vi "Debug_WFS_Tilt.vi"() -> ()   [LabVIEW 2014]
uses:
  AODAcq/AODAcq.lvclass
  <vilib>/rvi/interface/nirviReadWriteControl/nirviReadWriteControl.xnode
  FPGA_Control/AODRef.ctl
  <vilib>/DAQmx/write.llb/DAQmx Write (Analog DBL 1Chan 1Samp).vi
  <vilib>/Utility/file.llb/Write To Spreadsheet File (DBL).vi
  <vilib>/DAQmx/create/channels.llb/DAQmx Create Channel (AI-Voltage-Basic).vi
  <vilib>/DAQmx/read.llb/DAQmx Read (Analog 1D DBL NChan 1Samp).vi
  <vilib>/vision/driver/NI_Vision_Acquisition_Software.lvlib
  <vilib>/userdefined/High Color/IMAQdx.ctl
  <vilib>/vision/driver/IMAQdx.llb/IMAQdx Camera Control Mode.ctl
  <vilib>/rvi/errors/niLvFpgaAdjustHostInterfaceError.vi
  NiFpgaLv.dll
  <vilib>/Utility/error.llb/Error Cluster From Error Code.vi
  FPGA Bitfiles/AodScanner_FPGATarget_AODControl(FPGA)_TyJc9yYmyGA.lvbitx
panel:
  in  "Reps":i32=1
  out "Image":T1(plugin-control)
  in  "Measure centroid":bool
  out "Power":dbl
  in  "Save":bool
  in  "Range":dbl=214748364.8
  in  "stop":bool
  out "Corodinate Num":i32
  out "Num Coordinates":i32
  in  "NXHP":i32=10
  in  "NXLP":i32=10
  in  "NYHP":i32=10
  in  "NYLP":i32=10
  in  "Measure WFS":bool
  in  "Measure Power":bool
  in  "Hold time (ms)":u32=500
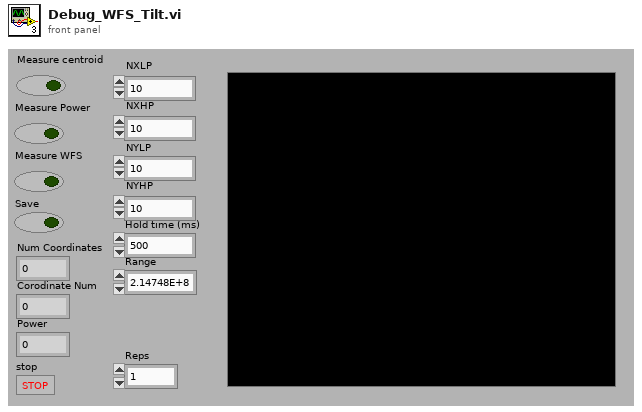
[diagram p1: front panel]
types:
  T1 = typedef "IMAQ Image.ctl" = refnum<image>
  T2 = typedef "NI_Vision_Acquisition_Software.lvlib/IMAQdx Camera Control Mode.ctl" = enum32{"Controller", "Listener"}
  T3 = typedef "IMAQdx.ctl" = refnum<k21>
  T4 = typedef "Image Type" = u32
  T5 = enum16{"Read", "Write", "ReadWrite", "BufferedRead", "BufferedReadWrite"}
  T6 = cluster{"XHP":i32, "XLP":i32, "YHP":i32, "YLP":i32}[]
  T7 = typedef "AODRef.ctl" = refnum<k20>
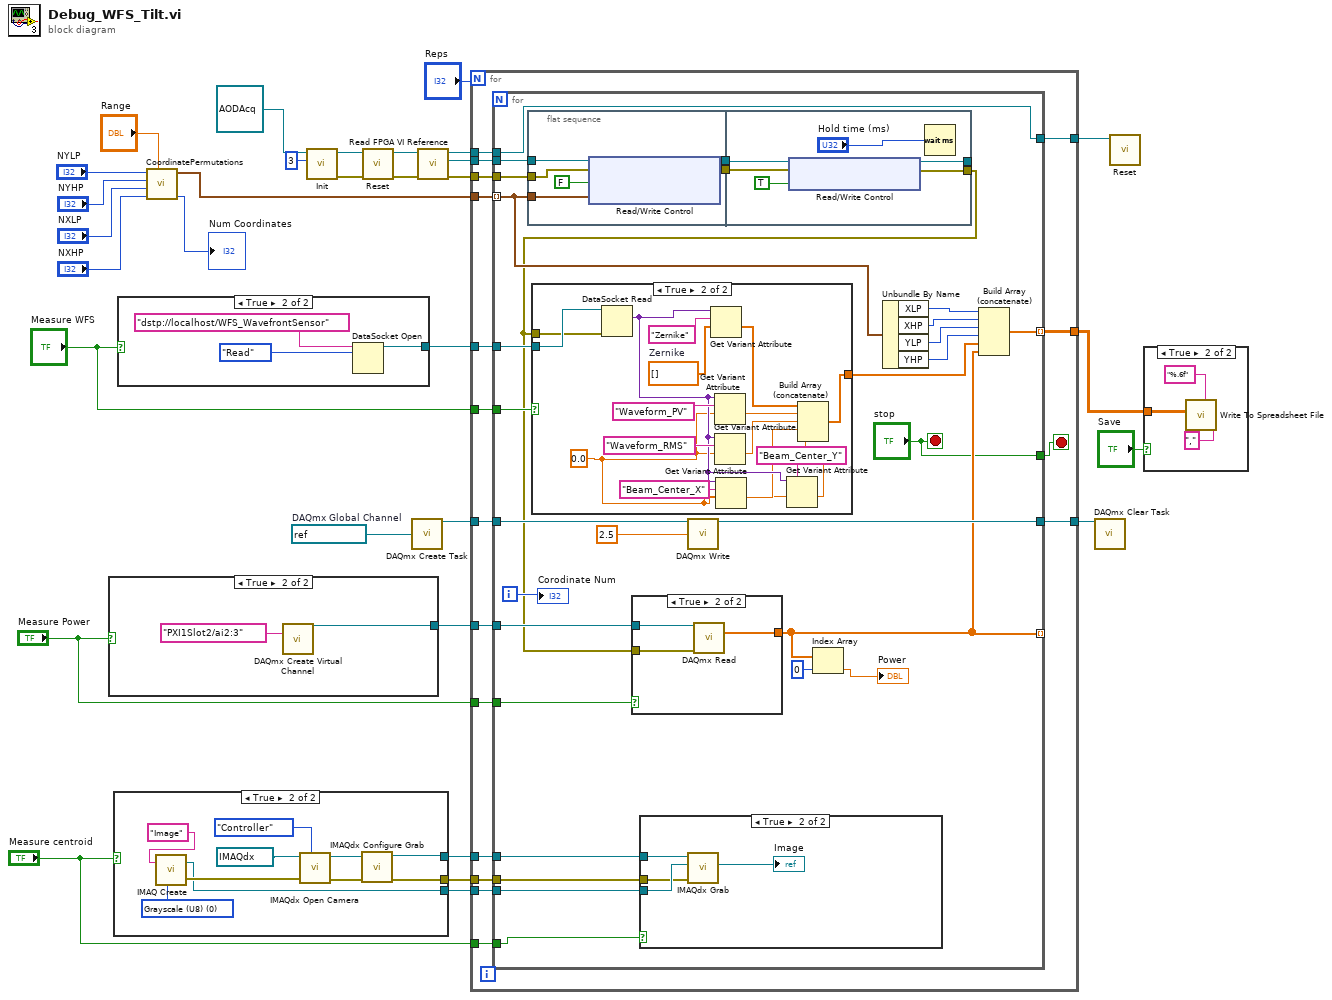
[diagram p0: block diagram]
diagram:
  w22 = refnum<k21> "AOD Gain"  # DAQmx Global Channel
  n1 = case shown="True" "Measure Power" {
    tunnel: [_ w32] -> w10
    frame False {
    }
    frame True {
      n2 = call-poly <vilib>:"DAQmx Create Virtual Channel.vi"("physical channels"=tag "PXI1Slot2/ai2:3") -> ("task out"=w32:refnum<k21>)  [unwired: 13 in, 1 out]
    }
  }
  n3 = case shown="True" "Measure centroid" {
    tunnel: [_ w35] -> w8
    tunnel: [_ w39] -> w6
    tunnel: [_ w34] -> w5
    frame False {
    }
    frame True {
      w41 = T4 0 items=["Grayscale (U8)", "Grayscale (I16)", "Grayscale (SGL)", "Complex (CSG)", "RGB (U32)", "HSL (U32)", "RGB (U64)", "Grayscale (U16)"] ("Image Type")
      n4 = call "IMAQ Create"("Image Name"="Image", "Image Type"=w41) -> ("New Image"=w39:T1, "error out"=w40:errorcluster)  [unwired: 3 in]
      n5 = call <vilib>:"IMAQdx Open Camera.vi"("Camera Control Mode"=IMAQdx_Camera_Control_Mode."Controller", "error in"=w40, "Session In"=T3 "cam1") -> ("error out"=w37:errorcluster, "Session Out"=w36:T3)  [unwired: 7 in]
      n6 = call <vilib>:"IMAQdx Configure Grab.vi"("error in"=w37, "Session In"=w36) -> ("error out"=w34:errorcluster, "Session Out"=w35:T3)  [unwired: 8 in]
    }
  }
  n7 = case shown="True" "Measure WFS" {
    tunnel: [_ w44] -> w23
    frame False {
    }
    frame True {
      n8 = DataSocket Open(10:T5."Read" ("mode"), 11:"dstp://localhost/WFS_WavefrontSensor" ("URL")) -> (3:w44:refnum<k13>)  [unwired: 2 in, 1 out]
    }
  }
  n9 = call "CoordinatePermutations.vi"("Range"="Range", "NXHP"="NXHP", "NXLP"="NXLP", "NYHP"="NYHP", "NYLP"="NYLP") -> ("Num Coordinates"=→"Num Coordinates":i32, "Coordinates"=w4:T6)  [unwired: 5 in]
  n10 = call-dynamic "Init.vi"("Channel"=i16 3, "AODAcq in"=refnum<class "AODAcq.lvclass"> refnum ("AODAcq.lvclass")) -> ("error out"=w29:errorcluster, "AODAcq out"=w30:refnum<class "AODAcq.lvclass">)  [unwired: 8 in]
  n11 = call-dynamic "Reset.vi"("error in (no error)"=w29, "AODAcq in"=w30) -> ("error out"=w26:errorcluster, "AODAcq out"=w28:refnum<class "AODAcq.lvclass">)  [unwired: 8 in]
  n12 = call <vilib>:"DAQmx Create Task.vi"("global virtual channels"=w22) -> ("task out"=w21:refnum<k21>)  [unwired: 4 in, 10 out]
  n13 = call-dynamic "Read FPGA VI Reference.vi"("error in (no error)"=w26, "AODAcq in"=w28) -> ("error out"=w25:errorcluster, "FPGA VI Reference"=w27:T7, "AODAcq out"=w19:refnum<class "AODAcq.lvclass">)  [unwired: 7 in]
  n14 = for {
    N: "Reps" -> [_]
    tunnel: w27 -> [w63]
    tunnel: w25 -> [w62]
    tunnel: "Measure WFS" -> [w61]
    tunnel: w23 -> [w60]
    tunnel: w21 -> [w59]
    tunnel: [w58] -> w20
    tunnel: w19 -> [w57]
    tunnel: [w56] -> w2
    tunnel: [w55] -> w12
    tunnel: w10 -> [w54]
    tunnel: "Measure Power" -> [w53]
    tunnel: w8 -> [w52]
    tunnel: "Measure centroid" -> [w51]
    tunnel: w6 -> [w50]
    tunnel: w5 -> [w49]
    tunnel: w4 -> [w48]
    stop <- w47 stop-if-true
    n15 = for {
      tunnel: w63 -> [w91]
      tunnel: w48 -> [w81] mode=indexing
      tunnel: w62 -> [w89]
      tunnel: w61 -> [w88]
      tunnel: w60 -> [w87]
      tunnel: w59 -> [w86]
      tunnel: [w84] -> w58
      tunnel: w57 -> [w83]
      tunnel: [w83] -> w56
      tunnel: [w75] -> w55 mode=indexing
      tunnel: w54 -> [w74]
      tunnel: w53 -> [w72]
      tunnel: [w71] -> _ mode=indexing
      tunnel: w52 -> [w67]
      tunnel: w51 -> [w68]
      tunnel: w50 -> [w66]
      tunnel: w49 -> [w65]
      tunnel: ["stop"] -> w47
      i -> [w82]
      stop <- "stop" stop-if-true
      n16 = flat-sequence {
        tunnel: w91 -> [w121]
        tunnel: [w119] -> w92
        tunnel: w81 -> [w118]
        tunnel: [w117] -> w90
        tunnel: w89 -> [w116]
        tunnel: w92 -> [w127]
        tunnel: w90 -> [w124]
        tunnel: [w123] -> w73
        tunnel: [w122] -> _
        frame #0 {
          n17 = xnode "Read/Write Control"("FPGA VI Reference In"=w121, "error in"=w116, "Debug.SetCoordinate"=FALSE, "Debug.Coordinate"=w118) -> ("FPGA VI Reference Out"=w119:T7, "error out"=w117:errorcluster)
        }
        frame #1 {
          n18 = xnode "Read/Write Control"("FPGA VI Reference In"=w127, "error in"=w124, "Debug.SetCoordinate"=TRUE) -> ("FPGA VI Reference Out"=w122:T7, "error out"=w123:errorcluster)
          n19 = Wait (ms)(milliseconds to wait="Hold time (ms)") -> ()  [unwired: 1 out]
        }
      }
      n20 = case shown="True" w88 {
        tunnel: w87 -> [_ w113]
        tunnel: w73 -> [_ w112]
        tunnel: [_ w106] -> w76
        frame False {
        }
        frame True {
          w101 = 0.0
          w115 = dbl[] []  # Zernike
          n21 = DataSocket Read(8:w112, 11:w113) -> (2:w105:variant)  [unwired: 3 in, 6 out]
          n22 = Get Variant Attribute(Variant=w105, name="Zernike", default value (empty Variant)=w115) -> (value=w109:dbl[])  [unwired: 1 in, 3 out]
          n23 = Get Variant Attribute(Variant=w105, name="Waveform_PV", default value (empty Variant)=w101) -> (value=w108:dbl)  [unwired: 1 in, 3 out]
          n24 = Get Variant Attribute(Variant=w105, name="Waveform_RMS", default value (empty Variant)=w101) -> (value=w107:dbl)  [unwired: 1 in, 3 out]
          n25 = Get Variant Attribute(Variant=w105, name="Beam_Center_X", default value (empty Variant)=w101) -> (value=w102:dbl)  [unwired: 1 in, 3 out]
          n26 = Get Variant Attribute(Variant=w105, name="Beam_Center_Y", default value (empty Variant)=w101) -> (value=w100:dbl)  [unwired: 1 in, 3 out]
          n27 = Build Array (concatenate)(w109, w108, w107, w102, w100) -> (w106:dbl[])
        }
      }
      n28 = case shown="True" w72 {
        tunnel: w74 -> [_ w99]
        tunnel: w73 -> [_ w98]
        tunnel: [_ w97] -> w71
        frame False {
        }
        frame True {
          n29 = call-poly <vilib>:"DAQmx Read.vi"("task/channels in"=w99, "error in"=w98) -> ("data"=w97:dbl[])  [unwired: 11 in, 2 out]
        }
      }
      n30 = case shown="True" w68 {
        tunnel: w67 -> [_ w96]
        tunnel: w66 -> [_ w94]
        tunnel: w65 -> [_ w93]
        frame False {
        }
        frame True {
          n31 = call <vilib>:"IMAQdx Grab.vi"("error in"=w93, "Image In"=w94, "Session In"=w96) -> ("Image Out"=→"Image":T1)  [unwired: 5 in, 3 out]
        }
      }
      n32 = call-poly <vilib>:"DAQmx Write.vi"("task/channels in"=w86, "data"=2.5) -> ("task out"=w84:refnum<k21>)  [unwired: 11 in, 2 out]
      n33 = Index Array(array=w71, index=0) -> (element=→"Power":dbl)
      n34 = Unbundle By Name(w81) -> ("XLP"=w80:i32, "XHP"=w79:i32, "YLP"=w78:i32, "YHP"=w77:i32)
      n35 = Build Array (concatenate)(w80, w79, w78, w77, w76, w71) -> (w75:dbl[])
      "Corodinate Num" <- w82
    }
  }
  n36 = call <vilib>:"DAQmx Clear Task.vi"("task in"=w20) -> ()  [unwired: 14 in, 1 out]
  n37 = call-dynamic "Reset.vi"("AODAcq in"=w2) -> ()  [unwired: 9 in, 2 out]
  n38 = case shown="True" "Save" {
    tunnel: w12 -> [_ w130]
    frame False {
    }
    frame True {
      n39 = call-poly <vilib>:"Write To Spreadsheet File.vi"("delimiter (\\t)"="," ("delimiter (\\t)"), "format (%.3f)"="%.6f", "2D data"=w130) -> ()  [unwired: 5 in, 1 out]
    }
  }
